vi "Save Configuration Settings to XML.vi"(8 "error in (no error)":errorcluster, 11 "User Configuration":T1={"Hardware Configuration"={"HW Refnum <Replace Me>"="", "Signal Type <Replace Me>"=enum."Sine Wave"}, "Analysis Configuration"={"Statistics"=TRUE}, "New Data Behavior"=enum."Replace"}) -> (0 "error out":errorcluster)   [LabVIEW 2023]
doc: "Saves the user-specified configuration data to an XML file. This is used to remember settings between executions."
uses:
  controls/User Specified Data.ctl
  controls/HW Configuration.ctl
  controls/Simulated Signal Type.ctl
  controls/Analysis Configuration.ctl
  controls/New Data Behavior.ctl
  <vilib>/Utility/xml.llb/Write to XML File(string).vi
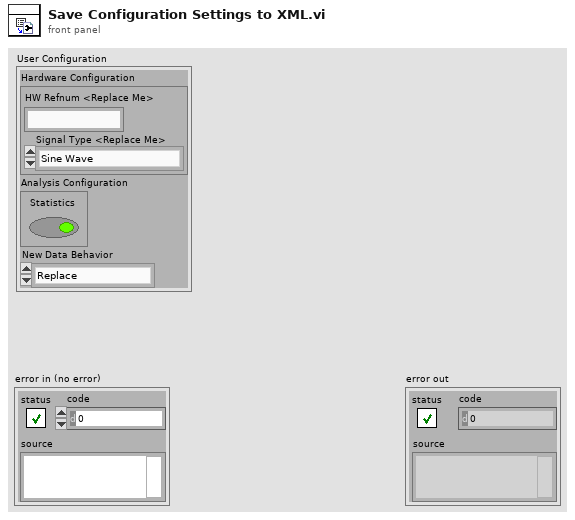
[diagram p1: front panel]
types:
  T1 = typedef "User Specified Data.ctl" = cluster{"Hardware Configuration":T2, "Analysis Configuration":T4, "New Data Behavior":T5}
  T2 = typedef "HW Configuration.ctl" = cluster{"HW Refnum <Replace Me>":string, "Signal Type <Replace Me>":T3}
  T3 = typedef "Simulated Signal Type.ctl" = enum16{"Sine Wave", "Square Wave"}
  T4 = typedef "Analysis Configuration.ctl" = cluster{"Statistics":bool}
  T5 = typedef "New Data Behavior.ctl" = enum16{"Replace", "Overlay", "Append"}
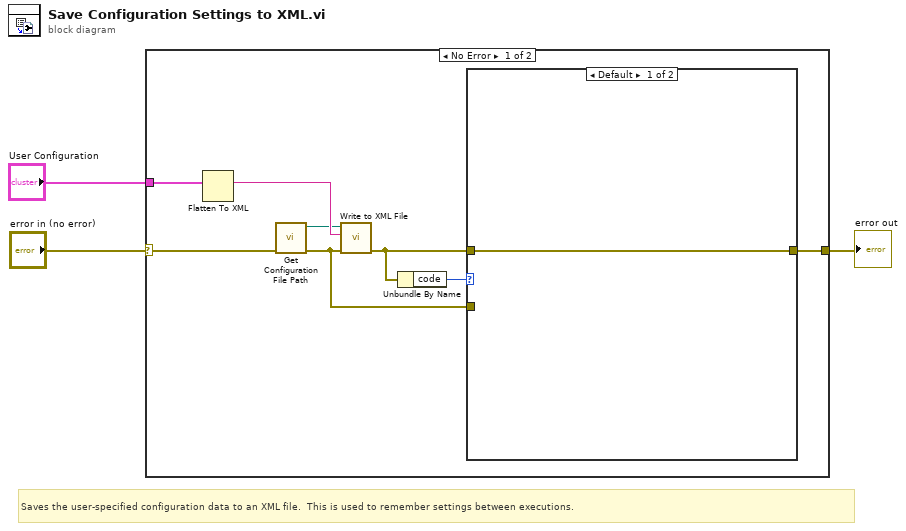
[diagram p0: block diagram]
diagram:
  # "Saves the user-specified configuration data to an XML file.  This is used to remember settings between executions."
  n1 = case shown="No Error" "error in (no error)" {
    selector: "error in (no error)" -> [w8 w14]
    tunnel: [w5 w14] -> w2
    tunnel: "User Configuration" -> [w11 _]
    frame No Error {
      n2 = Flatten To XML(6:w11) -> (2:w10:string)
      n3 = call "Get Configuration File Path.vi"("error in (no error)"=w8) -> ("error out"=w4:errorcluster, "XML File Path"=w9:path)  [unwired: 9 in]
      n4 = call-poly <vilib>:"Write to XML File.vi"("error in (no error)"=w4, "XML Input"=w10, "XML File Path"=w9) -> ("error out"=w6:errorcluster)  [unwired: 6 in, 2 out]
      n5 = Unbundle By Name(w6) -> ("code"=w7:i32)
      n6 = case shown="Default" w7 {
        tunnel: [w12 w13] -> w5
        tunnel: w6 -> [w12 _]
        tunnel: w4 -> [_ w13]
        frame Default {
        }
        frame 8 {
          # "Ignore a permissions error when attempting to save the Settings.xml file."
          # "#CodeRecommended - Add code here to perform additional actions if a permissions error occurs when saving the Settings.xml file."
        }
      }
    }
    frame Error {
    }
  }
  "error out" <- w2
